vi "Compile with Context.vi"(8 "Error In":errorcluster) -> (0 "Error Out":errorcluster)   [LabVIEW 2018, in "Tests.lvlib" / "Compile.lvlib"]
uses:
  Compile.lvlib
  src/Toolkit/Low-Level/Context/Compiler.lvclass
  src/Toolkit/Data/Map/Map.lvclass
  D:/Users/cfield/Code/Field R&D Services/Labstache/src/Toolkit/Data/Datum/Datum.lvclass
  src/Toolkit/Data/Map/Support/From String.vi
  src/Toolkit/Support/Compile with Data.vi
  <vilib>/addons/_JKI Toolkits/Caraya/classes/Test/Test.lvclass
  <vilib>/addons/_JKI Toolkits/Caraya/classes/Assert/Assert.lvclass
  src/Toolkit/Toolkit.lvlib
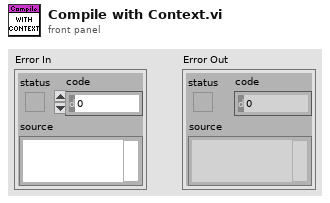
[diagram p1: front panel]
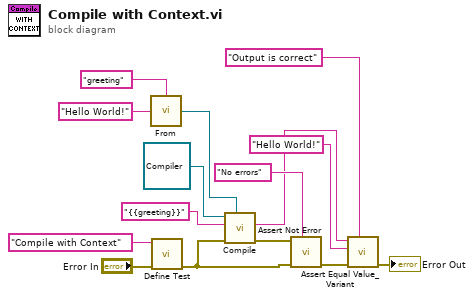
[diagram p0: block diagram]
diagram:
  n1 = call-poly "From.vi"("Value"="Hello World!", "Key"="greeting") -> ("Map"=w6:refnum<class "Map.lvclass">)
  n2 = call <vilib>:"Define Test.vi"("error in (no error)"="Error In", "Label (VI Title)"="Compile with Context") -> ("error out"=w3:errorcluster)  [unwired: 9 in]
  n3 = call-poly "Compile.vi"("Data"=w6, "Error In"=w3, "Input"="{{greeting}}" ("format string"), "Context In"=refnum<class "Compiler.lvclass"> refnum) -> ("Error Out"=w2:errorcluster, "Output"=w4:string)  [unwired: 5 in, 1 out]
  n4 = call <vilib>:"Assert Not Error.vi"("Label"="No errors", "error in (no error)"=w3, "Not Error?"=w2) -> ("error out"=w12:errorcluster)  [unwired: 8 in]
  n5 = call <vilib>:"Assert Equal Value_Variant.vi"("Label"="Output is correct", "error in (no error)"=w12, "Y"="Hello World!" ("Value"), "X"=w4) -> ("error out"=→"Error Out":errorcluster)  [unwired: 7 in]
